vi "Generic_error_logger.vi"(7 "clear error?":bool, 8 "Error to log":errorcluster) -> (0 "error or cleared error out":errorcluster)   [LabVIEW 2014]
doc: "this is VI documentation"
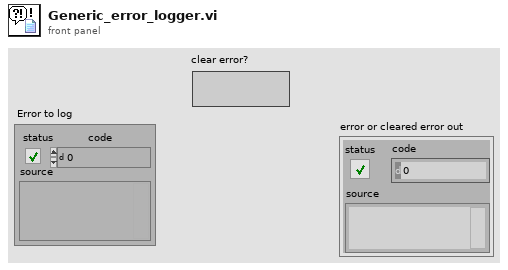
[diagram p1: front panel]
types:
  T1 = enum16{"open", "replace", "create", "open or create", "replace or create", "replace or create with confirmation"}
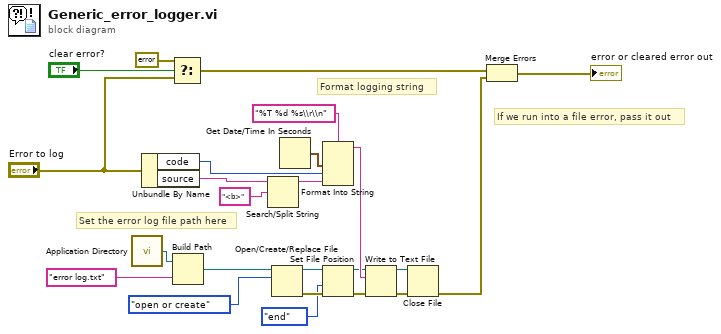
[diagram p0: block diagram]
diagram:
  # "Format logging string"
  # "If we run into a file error, pass it out"
  # "Set the error log file path here"
  n1 = call <vilib>:"Application Directory.vi"() -> ("Application Directory"=w14:path)
  n2 = Unbundle By Name("Error to log") -> ("code"=w21:i32, "source"=w24:string)
  n3 = Select(t=errorcluster {"status"=FALSE, "code"=0, "source"=""}, s="clear error?", f="Error to log") -> (s? t:f=w18:errorcluster)
  n4 = Build Path(base path=w14, name or relative path="error log.txt") -> (appended path=w12:path)
  n5 = Search/Split String(string=w24, search string/char (-)="<b>") -> (substring before match=w22:string)  [unwired: 1 in, 2 out]
  n6 = Open/Create/Replace File(file path (use dialog)=w12, operation (0:open)=T1."open or create") -> (refnum out=w10:refnum<file>, error out=w11:errorcluster)  [unwired: 4 in, 1 out]
  n7 = Get Date/Time In Seconds() -> (seconds since 1Jan1904=w20:timestamp)
  n8 = Format Into String(format string="%T %d %s\\r\\n", w20, w21, w22) -> (resulting string=w15:string)  [unwired: 2 in, 1 out]
  n9 = Set File Position(refnum=w10, from (0:start)=enum16{"start", "end", "current"}."end", error in=w11) -> (refnum out=w8:refnum<file>, error out=w7:errorcluster)  [unwired: 1 in]
  n10 = Write to Text File(file (use dialog)=w8, text=w15, error in=w7) -> (refnum out=w5:refnum<file>, error out=w6:errorcluster)  [unwired: 1 in, 1 out]
  n11 = Close File(refnum=w5, error in=w6) -> (error out=w3:errorcluster)  [unwired: 1 out]
  n12 = Merge Errors(w18, w3) -> (→"error or cleared error out":errorcluster)
